vi "DRIVE_SPEED_CONTROL.vi"(5 "Speed PID":T1, 6 "Speed (PV)":dbl, 9 "Speed Target (SP)":dbl, 10 "Max SP Rate":dbl, 11 "Max Speed Ft/Sec":dbl) -> (2 "SpeedDmd":dbl, 3 "CO-ControlOutput":dbl)   [LabVIEW 2019]
uses:
  <vilib>/Rock Robotics/WPI/ThirdParty/JAS_Junk/TrajLib/Trajectory_Library.lvlib
  DRIVE_PID_TUNING.ctl
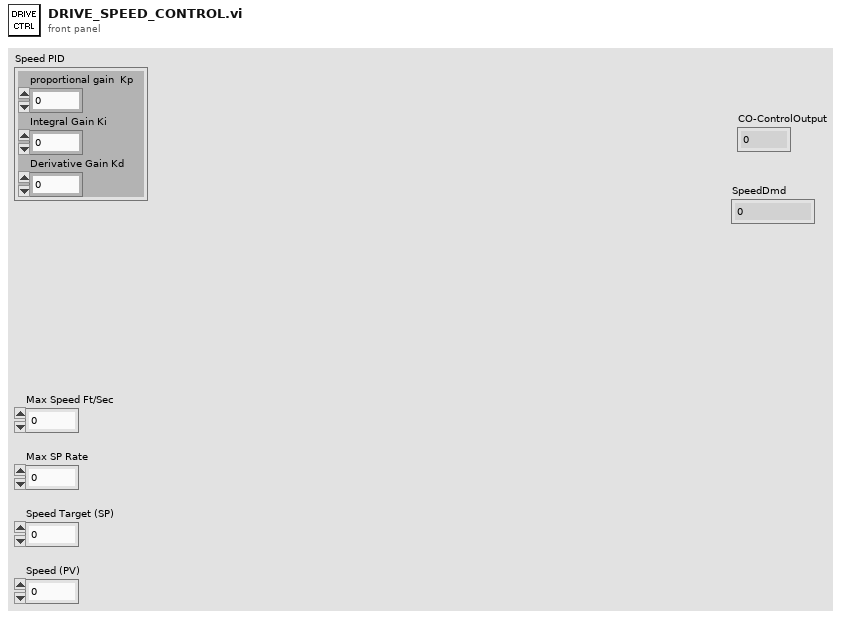
[diagram p1: front panel]
types:
  T1 = typedef "DRIVE_PID_TUNING.ctl" = cluster{"proportional gain  Kp":dbl, "Integral Gain Ki":dbl, "Derivative Gain Kd":dbl}
  T2 = typedef "Trajectory_Library.lvlib/PID_ADV_TUNING.ctl" = cluster{"Kf":dbl, "Kp":dbl, "Ki":dbl, "Kd":dbl, "MaximumIntegral":dbl, "MinimumIntegral":dbl, "Filter Derivative":bool}
  T3 = typedef "Trajectory_Library.lvlib/PID_ADV_LIMITS.ctl" = cluster{"MaxInput":dbl, "MinInput":dbl, "Continuous":bool, "MaxOutput":dbl, "MinOutput":dbl}
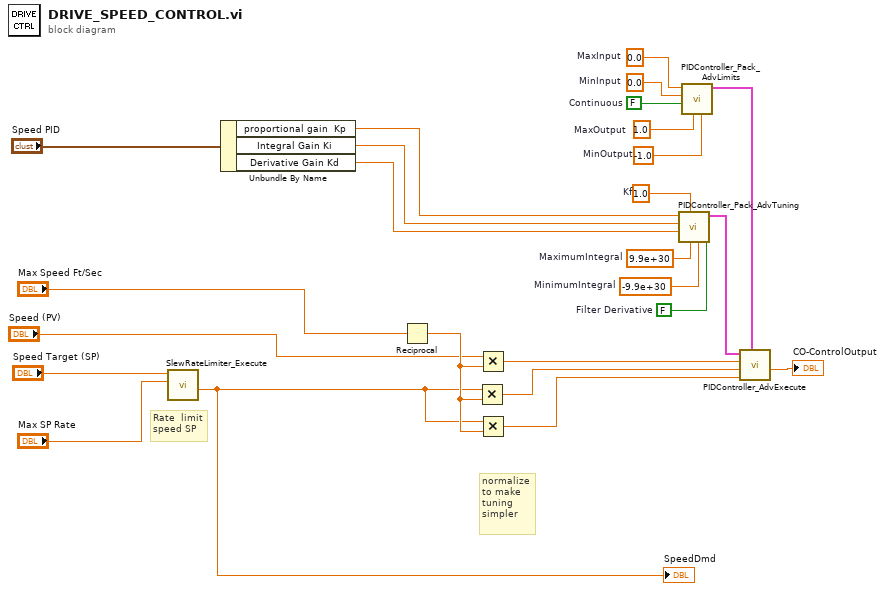
[diagram p0: block diagram]
diagram:
  w6 = 1.0  # Kf
  w7 = 9.9e+30  # MaximumIntegral
  w8 = -9.9e+30  # MinimumIntegral
  w9 = FALSE  # Filter Derivative
  w11 = 0.0  # MinInput
  w12 = FALSE  # Continuous
  w13 = 1.0  # MaxOutput
  w10 = -1.0  # MinOutput
  w14 = 0.0  # MaxInput
  # "Rate  limit\nspeed SP"
  # "normalize\nto make\ntuning\nsimpler"
  n1 = call <vilib>:"SlewRateLimiter_Execute.vi"("Rate"="Max SP Rate", "Input"="Speed Target (SP)") -> ("Output"=w1:dbl)  [unwired: 8 in, 1 out]
  "SpeedDmd" <- w1
  n2 = Unbundle By Name("Speed PID") -> ("proportional gain  Kp"=w22:dbl, "Integral Gain Ki"=w23:dbl, "Derivative Gain Kd"=w24:dbl)
  n3 = Reciprocal(x="Max Speed Ft/Sec") -> (1/x=w3:dbl)
  n4 = Multiply(x=w1, y=w3) -> (x*y=w18:dbl)
  n5 = Multiply(x="Speed (PV)", y=w3) -> (x*y=w21:dbl)
  n6 = Multiply(x=w1, y=w3) -> (x*y=w19:dbl)
  n7 = call <vilib>:"PIDController_Pack_AdvTuning.vi"("Filter Derivative"=w9, "MinimumIntegral"=w8, "MaximumIntegral"=w7, "Kf"=w6, "Kd"=w24, "Ki"=w23, "Kp"=w22) -> ("Adv PID Tuning"=w15:T2)  [unwired: 4 in]
  n8 = call <vilib>:"PIDController_Pack_AdvLimits.vi"("MinOutput"=w10, "MaxOutput"=w13, "Continuous"=w12, "MinInput"=w11, "MaxInput"=w14) -> ("Adv PID Limits"=w16:T3)  [unwired: 6 in]
  n9 = call <vilib>:"PIDController_AdvExecute.vi"("Adv PID Limits"=w16, "FF-FeedForward"=w19, "SP-SetPoint"=w18, "PV-Measurement"=w21, "Adv PID Tuning"=w15) -> ("CO-ControlOutput"=→"CO-ControlOutput":dbl)  [unwired: 4 in, 2 out]
